vi "uA_DAQ_Init_Monitor_Stream_vbat.vi"(8 "error in (no error)":errorcluster, 9 "Sample rate":u32=20000, 11 "USB":tag) -> (0 "error out":errorcluster, 3 "Refnum out":refnum<k21>)   [LabVIEW 2017]
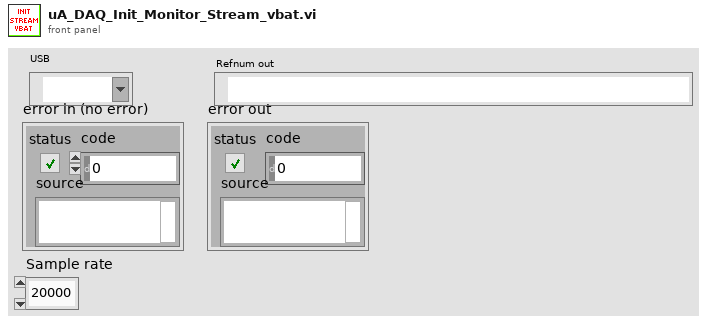
[diagram p1: front panel]
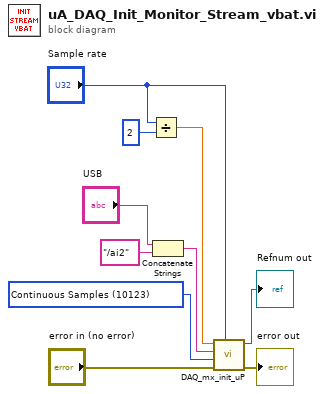
[diagram p0: block diagram]
diagram:
  w8 = 10123 items=["Finite Samples"=10178, "Continuous Samples"=10123, "Hardware Timed Single Point"=12522] ("sample mode")
  n1 = Divide(x="Sample rate", y=u32 2) -> (x/y=w1:dbl)
  n2 = Concatenate Strings("USB", "/ai2" ("ADC_Ch")) -> (w7:string)
  n3 = call "DAQ_mx_init_uP.vi"("rate"="Sample rate", "error in"="error in (no error)", "sample mode"=w8, "physical channel"=w7, "number of samples"=w1) -> ("error out"=→"error out":errorcluster, "task out"=→"Refnum out":refnum<k21>)  [unwired: 5 in]
